vi "TrackingComm.vi"(2 "error in (no error)":errorcluster, 3 "OWL Freq Hz(default: 480)":dbl=480.0 format="%.1f", 4 "marker tally (default: 32)":i32=32, 5 "server address":string="192.168.0.101") -> (0 "error out":errorcluster, 1 "connected to server?":bool)   [LabVIEW 2011]
uses:
  ctrInitFlags.ctl
  ctrCommonFlags.ctl
  ctrTrackersFlags.ctl
  ctrMarkersFlags.ctl
  ctrSetsFlags.ctl
  C:/Program Files/Phasespace/libowlsock.dll
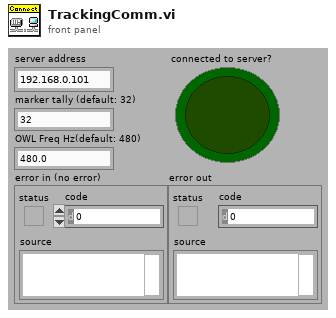
[diagram p1: front panel]
types:
  T1 = typedef "ctrInitFlags.ctl" = u16
  T2 = typedef "ctrCommonFlags.ctl" = u16
  T3 = typedef "ctrTrackersFlags.ctl" = u16
  T4 = typedef "ctrMarkersFlags.ctl" = u16
  T5 = typedef "ctrSetsFlags.ctl" = u16
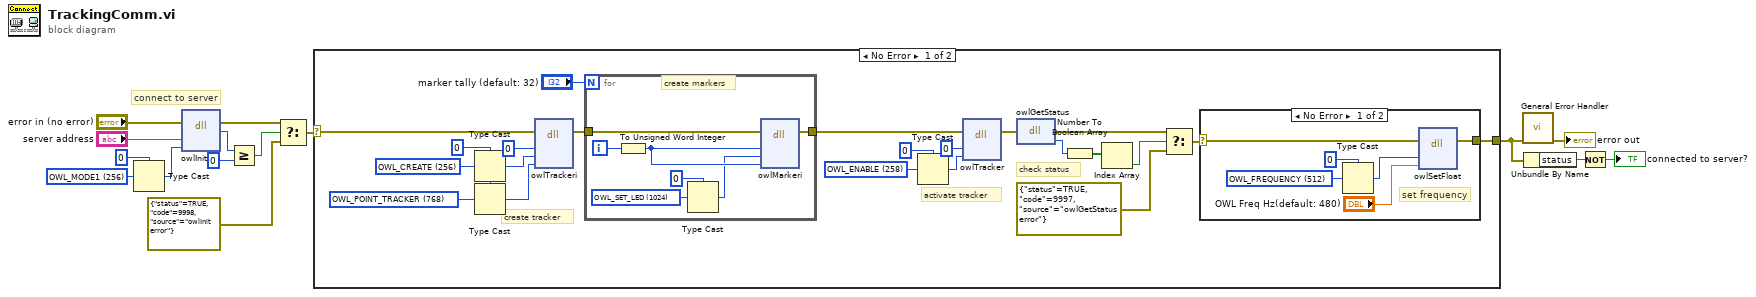
[diagram p0: block diagram]
diagram:
  w4 = T1 256 items=["OWL_SLAVE"=1, "OWL_FILE"=2, "OWL_POSTPROCESS"=16, "OWL_MODE1"=256, "OWL_MODE2"=512, "OWL_MODE3"=768, "OWL_MODE4"=1024, "OWL_LASER"=2560, "OWL_CALIB"=3072, "OWL_CALIBPLANAR"=3840]
  # "connect to server"
  n1 = Type Cast(type=u16 0, x=w4) -> (*(type *) &x=w3:u16)
  n2 = dll-call lib="C:/Program Files/Phasespace/libowlsock.dll" fn="owlInit"(error in="error in (no error)", "server"="server address", "flags"=w3) -> (error out=w10:errorcluster, "return type"=w14:i16)  [unwired: 4 in, 1 out]
  n3 = Greater Or Equal?(x=w14, y=i16 0) -> (x >= y?=w11:bool)
  n4 = Select(t=w10, s=w11, f=errorcluster {"status"=TRUE, "code"=9998, "source"="owlInit error"} ("error out")) -> (s? t:f=w9:errorcluster)
  n5 = case shown="No Error" w9 {
    selector: w9 -> [w36 w52]
    tunnel: [w37 w52] -> w7
    frame No Error {
      w20 = T2 258 items=["OWL_CREATE"=256, "OWL_DESTROY"=257, "OWL_ENABLE"=258, "OWL_DISABLE"=259] ("Common flages")
      w23 = T3 768 items=["OWL_POINT_TRACKER"=768, "OWL_RIGID_TRACKER"=769]
      w22 = u16 0 ("y")
      w26 = T2 256 items=["OWL_CREATE"=256, "OWL_DESTROY"=257, "OWL_ENABLE"=258, "OWL_DISABLE"=259] ("Common flages")
      # "activate tracker"
      # "create tracker"
      # "check status"
      n6 = Type Cast(type=w22, x=w26) -> (*(type *) &x=w25:u16)
      n7 = Type Cast(type=w22, x=w23) -> (*(type *) &x=w24:u16)
      n8 = dll-call lib="C:/Program Files/Phasespace/libowlsock.dll" fn="owlTrackeri"(error in=w36, "tracker"=u16 0 ("y"), "pname"=w25, "param"=w24) -> (error out=w32:errorcluster)  [unwired: 5 in, 2 out]
      n9 = for {
        N: "marker tally (default: 32)" -> [_]
        tunnel: w32 -> [w43]
        tunnel: [w42] -> w33
        i -> [w44]
        w40 = T4 1024 items=["OWL_SET_LED"=1024, "OWL_SET_POSITION"=1025, "OWL_CLEAR_MARKER"=1026]
        # "create markers"
        n10 = To Unsigned Word Integer(number=w44) -> (unsigned 16bit integer=w41:u16)
        n11 = Type Cast(type=u16 0 ("y"), x=w40) -> (*(type *) &x=w39:u16)
        n12 = dll-call lib="C:/Program Files/Phasespace/libowlsock.dll" fn="owlMarkeri"(error in=w43, "marker"=w41, "pname"=w39, "param"=w41) -> (error out=w42:errorcluster)  [unwired: 5 in, 2 out]
      }
      n13 = Type Cast(type=u16 0 ("y"), x=w20) -> (*(type *) &x=w19:u16)
      n14 = dll-call lib="C:/Program Files/Phasespace/libowlsock.dll" fn="owlTracker"(error in=w33, "tracker"=u16 0, "pname"=w19) -> (error out=w35:errorcluster)  [unwired: 4 in, 2 out]
      n15 = dll-call lib="C:/Program Files/Phasespace/libowlsock.dll" fn="owlGetStatus"(error in=w35) -> (error out=w29:errorcluster, "return type"=w18:u16)  [unwired: 2 in, 1 out]
      n16 = Number To Boolean Array(number=w18) -> (Boolean array=w17:bool[])
      n17 = Index Array(array=w17) -> (element=w16:bool)  [unwired: 1 in]
      n18 = Select(t=w29, s=w16, f=errorcluster {"status"=TRUE, "code"=9997, "source"="owlGetStatus error"} ("error out")) -> (s? t:f=w28:errorcluster)
      n19 = case shown="No Error" w28 {
        selector: w28 -> [w50 w51]
        tunnel: [w49 w51] -> w37
        frame No Error {
          w46 = T5 512 items=["OWL_FREQUENCY"=512, "OWL_STREAMING"=513, "OWL_INTERPOLATION"=514, "OWL_BUTTONS"=528, "OWL_MARKERS"=529, "OWL_RIGIDS"=530, "OWL_COMMDATA"=544, "OWL_TIMESTAMP"=545, "OWL_PLANES"=672, "OWL_DETECTORS"=673, "OWL_IMAGES"=674, "OWL_TRANSFORM"=49664]
          # "set frequency"
          n20 = Type Cast(type=u16 0 ("y"), x=w46) -> (*(type *) &x=w47:u16)
          n21 = dll-call lib="C:/Program Files/Phasespace/libowlsock.dll" fn="owlSetFloat"(error in=w50, "pname"=w47, "param"="OWL Freq Hz(default: 480)") -> (error out=w49:errorcluster)  [unwired: 4 in, 2 out]
        }
        frame Error {
        }
      }
    }
    frame Error {
    }
  }
  n22 = call <vilib>:"General Error Handler.vi"("error in (no error)"=w7) -> ("error out"=→"error out":errorcluster)  [unwired: 2 in, 12 out]
  n23 = Unbundle By Name(w7) -> ("status"=w6:bool)
  n24 = Not(x=w6) -> (.not. x?=→"connected to server?":bool)
